vi "Format Connection UI to Connection.vi"(10 "Modules and Connections":T1[](array[typedef]), 11 "Connection UI":T3) -> (3 "Connection":T3)   [LabVIEW 2017, in "Routing and Faulting System Explorer.lvlib"]
uses:
  Routing and Faulting System Explorer.lvlib
  Shared/Connection.ctl
  Possible Connections.ctl
  Shared/Routing and Faulting Hardware API/Types/Possible Connections for Endpoint.ctl
  Shared/Routing and Faulting Shared.lvlib
  Shared/Routing and Faulting Hardware API/Routing and Faulting Hardware API.lvlib
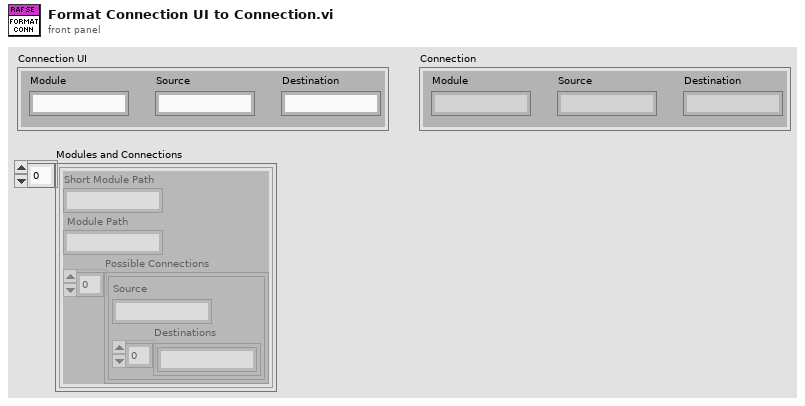
[diagram p1: front panel]
types:
  T1 = typedef "Routing and Faulting System Explorer.lvlib/Possible Connections.ctl" = cluster{"Short Module Path":string, " Module Path":string, "Possible Connections":T2[]}
  T2 = typedef "Routing and Faulting Hardware API.lvlib/Possible Connections for Endpoint.ctl" = cluster{"Source":string, "Destinations":string[]}
  T3 = typedef "Routing and Faulting Shared.lvlib/Connection.ctl" = cluster{"Module":string, "Source":string, "Destination":string}
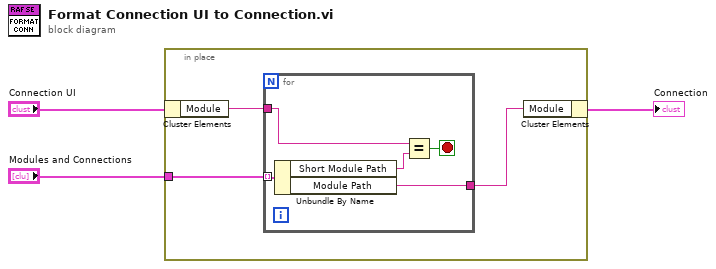
[diagram p0: block diagram]
diagram:
  n1 = in-place {
    in-place-border: "Modules and Connections" -> [w6]
    n2 = in-place-cluster #1("Connection UI") -> ("Module"=w5:string)
    n3 = for {
      tunnel: w6 -> [w11] mode=indexing
      tunnel: w5 -> [w9]
      tunnel: [w7] -> w4
      stop <- w8 stop-if-true
      n4 = Unbundle By Name(w11) -> ("Short Module Path"=w10:string, "Module Path"=w7:string)
      n5 = Equal?(x=w9, y=w10) -> (x = y?=w8:bool)
    }
    n6 = in-place-cluster #1("Module"=w4) -> (→"Connection":T3)
  }
